vi "Start.vi"(8 "error in":errorcluster, 11 "reference in":refnum<class "Instrument.lvclass">) -> (0 "error out":errorcluster, 3 "reference out":refnum<class "Instrument.lvclass">)   [LabVIEW 2023, in "HAL GOOP4.lvlib" / "Instrument.lvclass"]
uses:
  Instrument.lvclass
  Interfaces/IConfigure/IConfigure.lvclass
  Instrument.lvclass/Instrument.ctl
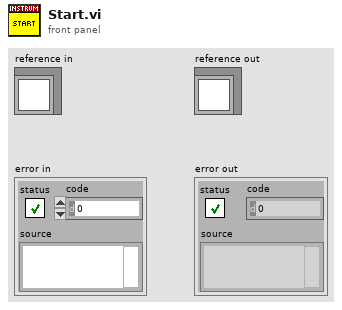
[diagram p1: front panel]
types:
  T1 = typedef "HAL GOOP4.lvlib/Instrument.lvclass/ObjectAttributes.ctl" = cluster{"IConfigure":refnum<class "IConfigure.lvclass">, "Ref Count":i16, "Start Count":i16}
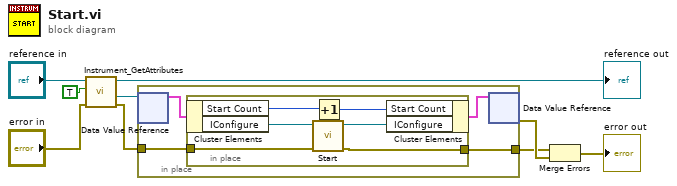
[diagram p0: block diagram]
diagram:
  n1 = call "Instrument_GetAttributes.vi"("Error In"="error in", "OnlyGetDvrReference(False)"=TRUE, "reference in"="reference in") -> ("Error Out"=w3:errorcluster, "DataRef"=w4:refnum<data-value>, "reference out"=→"reference out":refnum<class "Instrument.lvclass">)  [unwired: 5 in, 1 out]
  n2 = in-place {
    in-place-border: w3 -> [w11]
    in-place-border: [w10] -> w2
    n3 = in-place-dvr #1(w4) -> (w13:T1)  [unwired: 1 out]
    n4 = in-place {
      in-place-border: w11 -> [w17]
      in-place-border: [w16] -> w10
      n5 = in-place-cluster #2(w13) -> ("Start Count"=w15:i16, "IConfigure"=w19:refnum<class "IConfigure.lvclass">)
      n6 = call-dynamic "Start.vi"("error in (no error)"=w17, "IConfigure in"=w19) -> ("error out"=w16:errorcluster, "IConfigure out"=w18:refnum<class "IConfigure.lvclass">)  [unwired: 8 in]
      n7 = Increment(x=w15) -> (x+1=w14:i16)
      n8 = in-place-cluster #2("Start Count"=w14, "IConfigure"=w18) -> (w12:T1)
    }
    n9 = in-place-dvr #1(w12) -> (w5:errorcluster)  [unwired: 1 out]
  }
  n10 = Merge Errors(w2, w5) -> (→"error out":errorcluster)
